vi "RTD_save_preset_dialog.vi"(8 "error in":errorcluster, 11 "preset":T1 {"tref" format="%.3f"; "Rref [Ohm]" format="%.3f"; "RTD poly" format="%_6e"}) -> (0 "error out":errorcluster)   [LabVIEW 2020]
uses:
  RTD_preset.ctl
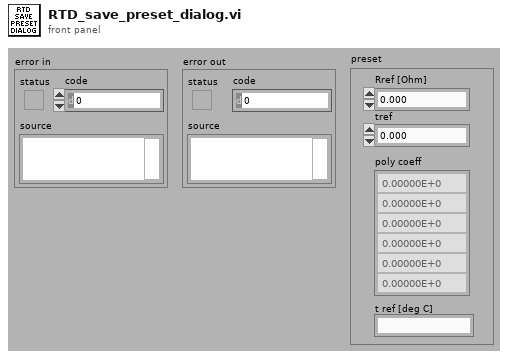
[diagram p1: front panel]
types:
  T1 = typedef "RTD_preset.ctl" = cluster{"Rref [Ohm]":dbl, "tref":dbl, "RTD poly":dbl[], "name":string}
  T2 = enum16{"open", "replace", "create", "open or create", "replace or create", "replace or create with confirmation"}
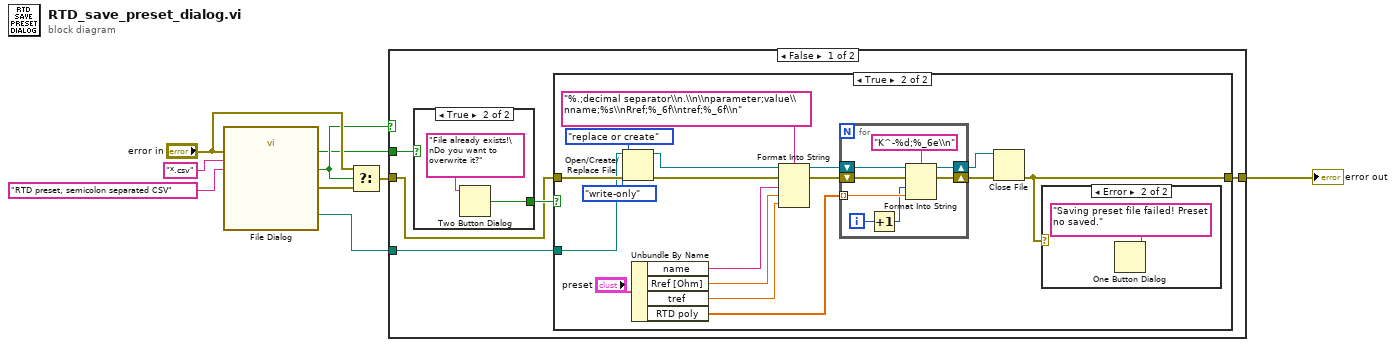
[diagram p0: block diagram]
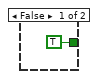
[diagram p4: hidden frame]
diagram:
  n1 = call "File Dialog"("error in"="error in", "pattern (all files)"="*.csv", "pattern label"="RTD preset, semicolon separated CSV") -> ("selected path"=w4:path, "exists"=w5:bool, "cancelled"=w7:bool, "error out"=w9:errorcluster)  [unwired: 9 in]
  n2 = Select(t="error in", s=w7, f=w9) -> (s? t:f=w6:errorcluster)
  n3 = case shown="False" w7 {
    tunnel: w6 -> [w12 w45]
    tunnel: w5 -> [w14 _]
    tunnel: w4 -> [w11 _]
    tunnel: [w10 w45] -> w3
    frame False {
      n4 = case shown="True" w14 {
        tunnel: [TRUE ("T button?") w43] -> w13
        frame False {
        }
        frame True {
          n5 = Two Button Dialog(message="File already exists!\nDo you want to overwrite it?") -> (T button?=w43:bool)  [unwired: 2 in]
        }
      }
      n6 = case shown="True" w13 {
        tunnel: w12 -> [w15 w32]
        tunnel: w11 -> [_ w31]
        tunnel: [w15 w18] -> w10
        frame False {
        }
        frame True {
          n7 = Open/Create/Replace File(file path (use dialog)=w31, error in=w32, operation (0:open)=T2."replace or create", access (0:read/write)=enum16{"read/write", "read-only", "write-only"}."write-only") -> (refnum out=w26:refnum<file>, error out=w28:errorcluster)  [unwired: 2 in, 1 out]
          n8 = Unbundle By Name("preset") -> ("name"=w24:string, "Rref [Ohm]"=w23:dbl, "tref"=w16:dbl, "RTD poly"=w17:dbl[])
          n9 = Format Into String(format string="%.;decimal separator\\n.\\n\\nparameter;value\\nname;%s\\nRref;%_6f\\ntref;%_6f\\n", initial string=w26, error in=w28, w24, w23, w16) -> (resulting string=w21:refnum<file>, error out=w22:errorcluster)
          n10 = for {
            tunnel: w17 -> [w39] mode=indexing
            shift-right: [w36] -> w20
            shift-left: w22 -> [w41]
            shift-right: [w37] -> w19
            shift-left: w21 -> [w40]
            i -> [w35]
            n11 = Increment(x=w35) -> (x+1=w34:i32)
            n12 = Format Into String(format string="K^-%d;%_6e\\n", initial string=w40, error in=w41, w34, w39) -> (resulting string=w37:refnum<file>, error out=w36:errorcluster)
          }
          n13 = Close File(refnum=w19, error in=w20) -> (error out=w18:errorcluster)  [unwired: 1 out]
          n14 = case shown="Error" w18 {
            frame No Error {
            }
            frame Error {
              n15 = One Button Dialog(message="Saving preset file failed! Preset no saved.") -> ()  [unwired: 1 in, 1 out]
            }
          }
        }
      }
    }
    frame True {
    }
  }
  "error out" <- w3
